vi "Enable Sessions.vi"(8 "error in (no error)":errorcluster, 10 "Session Implementation":refnum<class "Session.lvclass">, 11 "Server in":refnum<class "Server.lvclass">) -> (0 "error out":errorcluster, 3 "Server out":refnum<class "Server.lvclass">)   [LabVIEW 2020, in "HTTP Server.lvlib" / "Server.lvclass"]
doc: "Enables sessions in the webserver by providing a configured session implementation. The included implementation, available via Init File Storage.vi, saves session data based on randomly generated user cookies in a specified folder on disk. Sessions are specified by an Interface so it is possible to provide custom implementations that provide different storage mechanisms such as a different file format, SQLite, or some other way to persist session data across requests.\n\nOnce a session implementation is specified, handlers are automatically added to the processing to restore session values from the implementation based on a cookie session ID and to persist the session data via the implementation and send the session cookie as necessary in the response."
uses:
  Server.lvclass
  Session/Session.lvclass
  Server.lvclass/Server.ctl
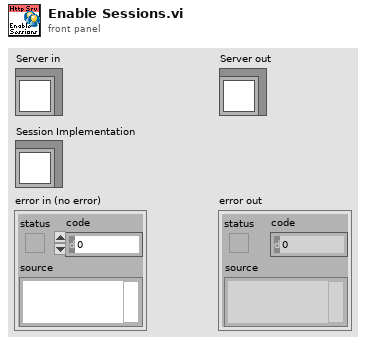
[diagram p1: front panel]
types:
  T1 = typedef "HTTP Server.lvlib/Server.lvclass/Ref Data.ctl" = cluster{"Connection Handler Map":T2, "Request Handler Map":T4, "Route Handler Map":T5, "Controller Handler Map":T6, "Controller Map":T7, "Response Handler Map":T8, "Complete Handler Map":T9, "Exception Handler Map":T10, "Connection Handler Index":u16, "Request Handler Index":u16, "Route Handler Index":u16, "Controller Handler Index":u16, "Controller Index":u16, "Response Handler Index":u16, "Complete Handler Index":u16, "Exception Handler Index":u16, "Values":refnum<class "Values.lvclass">, "Path":path, "Session Type":refnum<class "Session.lvclass">, "Session Cookie Name":string, "WebSocket Handler":refnum<class "WebSocket Handler.lvclass">, "WebSocket Handling":bool}
  T2 = typedef "HTTP Server.lvlib/Connection Handler Map.ctl" = map{T3, refnum<class "Connection Handler.lvclass">}
  T3 = typedef "HTTP Server.lvlib/Priority.ctl" = cluster{"Entity":u16, "Index":u16}
  T4 = typedef "HTTP Server.lvlib/Request Handler Map.ctl" = map{T3, refnum<class "Request Handler.lvclass">}
  T5 = typedef "HTTP Server.lvlib/Route Handler Map.ctl" = map{T3, refnum<class "Route Handler.lvclass">}
  T6 = typedef "HTTP Server.lvlib/Controller Handler Map.ctl" = map{T3, refnum<class "Controller Handler.lvclass">}
  T7 = typedef "HTTP Server.lvlib/Controller Map.ctl" = map{T3, refnum<class "Controller.lvclass">}
  T8 = typedef "HTTP Server.lvlib/Response Handler Map.ctl" = map{T3, refnum<class "Response Handler.lvclass">}
  T9 = typedef "HTTP Server.lvlib/Complete Handler Map.ctl" = map{T3, refnum<class "Complete Handler.lvclass">}
  T10 = typedef "HTTP Server.lvlib/Exception Handler Map.ctl" = map{T3, refnum<class "Exception Handler.lvclass">}
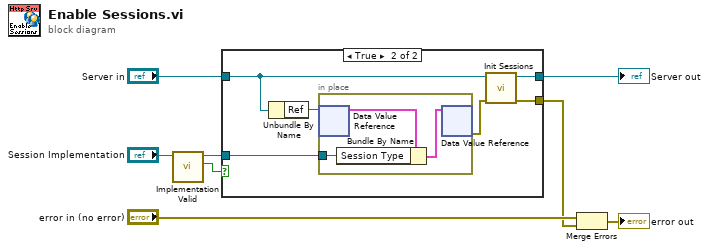
[diagram p0: block diagram]
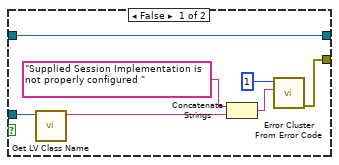
[diagram p2: hidden frame]
diagram:
  n1 = call "Implementation Valid.vi"("Session in"="Session Implementation") -> ("Valid?"=w2:bool, "Session out"=w1:refnum<class "Session.lvclass">)  [unwired: 8 in, 1 out]
  n2 = case shown="True" w2 {
    tunnel: "Server in" -> [w15 w20]
    tunnel: [w15 w18] -> w6
    tunnel: [w12 w17] -> w4
    tunnel: w1 -> [w13 w16]
    frame False {
      n3 = call <vilib>:"Get LV Class Name.vi"("object"=w13) -> ("class name"=w10:string)  [unwired: 9 in, 1 out]
      n4 = Concatenate Strings("Supplied Session Implementation is not properly configured " ("error message (\"\")"), w10) -> (w9:string)
      n5 = call <vilib>:"Error Cluster From Error Code.vi"("error message (\"\")"=w9, "error code (0)"=1) -> ("error out"=w12:errorcluster)  [unwired: 7 in]
    }
    frame True {
      n6 = Unbundle By Name(w20) -> ("Ref"=w21:refnum<data-value>)
      n7 = in-place {
        in-place-border: w16 -> [w22]
        n8 = in-place-dvr #1(w21) -> (w24:T1)  [unwired: 1 out]
        n9 = Bundle By Name(cluster=w24, "Session Type"=w22) -> (w23:T1)
        n10 = in-place-dvr #1(w23) -> (w19:errorcluster)  [unwired: 1 out]
      }
      n11 = call "Init Sessions.vi"("error in (no error)"=w19, "Server in"=w20) -> ("error out"=w17:errorcluster, "Server out"=w18:refnum<class "Server.lvclass">)  [unwired: 8 in]
    }
  }
  "Server out" <- w6
  n12 = Merge Errors("error in (no error)", w4) -> (→"error out":errorcluster)
